vi "Set Backpressure.vi"(6 "Direction":T1, 7 "init":bool, 8 "error in (no error)":errorcluster, 11 "Stand in":refnum<class "Stand.lvclass">) -> (0 "error out":errorcluster, 2 "done":bool, 3 "Stand out":refnum<class "Stand.lvclass">)   [LabVIEW 2019, in "Stand.lvclass"]
uses:
  Stand.lvclass
  D:/GIT H4000/H4000/src/Device_class/Device.lvclass
  TypeDef/Direction.ctl
  TypeDef/SP_TYPE.ctl
  Stand.lvclass/Stand.ctl
  TypeDef/State - BackPressure.ctl
  Valve Mode.ctl
  Device_class/Device.lvclass/Device.ctl
  AI_class/AI.lvclass/AI.ctl
  AnalogComparator_class/AnalogComparator.lvclass/AnalogComparator.ctl
  FPGA/TypeDef/DO index.ctl
  628d624b-520a-41e0-a7db-5fb9c9a9f1d4.vi
  Valve State Mode.vi
  AnalogComparator_class/GetStatus.vi
  Valve State Mode.vi/810e184e-eeb6-4027-a8ae-1422f3ce3d45.vi
  Valve State Mode.vi/57bd4a65-f3dc-44f5-8d68-677c2a197570.vi
  Valve State Mode.vi/03b2f9e4-fceb-4725-9b90-3fd10082a088.vi
  Valve State Mode.vi/3d0d09bd-48e8-482f-b1e2-a36b2bb65234.vi
  Valve State Mode.vi/33d3f26a-dc4a-4f56-bf0a-61d04c5d7434.vi
  Valve State Mode.vi/52af9d47-24d1-4057-80bf-8d93bfb3d17d.vi
  Valve State Mode.vi/094228cb-a119-423c-9af8-5a16f059a318.vi
  Valve State Mode.vi/bf5ad1e6-a0ae-4579-ad74-ca8f304cb7cf.vi
  Valve State Mode.vi/eb4d2b76-f0f0-4e1d-bda0-609c5f37b4e7.vi
  Const All Valve.vi
  Global/Global Constant.vi
  FPGA_API_class/FPGA API.lvclass
  Device_class/Device.lvclass
  AI_class/AI.lvclass
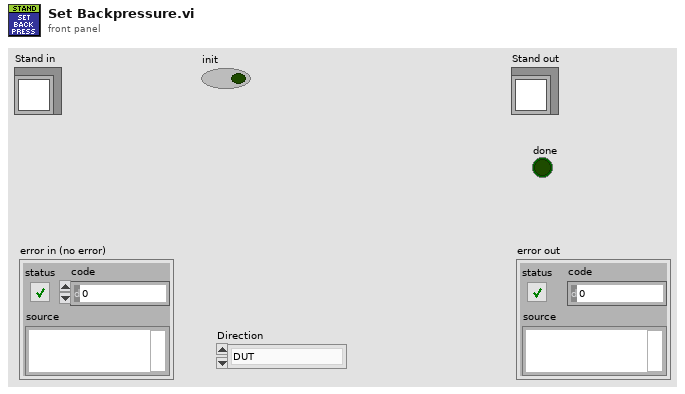
[diagram p1: front panel]
types:
  T1 = typedef "Direction.ctl" = enum8{"DUT", "Chamber"}
  T2 = typedef "SP_TYPE.ctl" = enum16{"ERROR", "ZIRO", "BASE", "SP"}
  T3 = typedef "State - BackPressure.ctl" = enum16{"Check", "Close Inlet", "Open 33_7", "Open Inlet", "Wait", "Close Inlet 2"}
  T4 = typedef "Valve Mode.ctl" = enum16{"Filling DUT", "Filling Chamber", "Pump Pressure DUT", "Pump Pressure Chamber", "Haskel Pressure DUT", "Haskel Pressure Chamber", "Slow Release DUT", "Slow Release Chamber", "Fast Release DUT", "Fast Release Chamber", "Fast Release DUT and Chamber", "Leak Pressure DUT", "Leak Pressure Chamber", "Back Pressure DUT", "Back Pressure Chamber", "Fully Closed", "Drain", "Block DUT", "Block Chamber"}
  T5 = typedef "DO index.ctl" = u8
  T6 = typedef "AI_Data.ctl" = cluster{"Stat Data":T7, "OutOfRangeMax":bool, "OutOfRangeMin":bool, "HIHI":bool, "HI":bool, "LO":bool, "LOLO":bool}
  T7 = typedef "AI Statistics Data.ctl" = cluster{"raw mean":dbl, "scl mean":dbl, "raw mean 1Hz":dbl, "scl mean 1Hz":dbl}
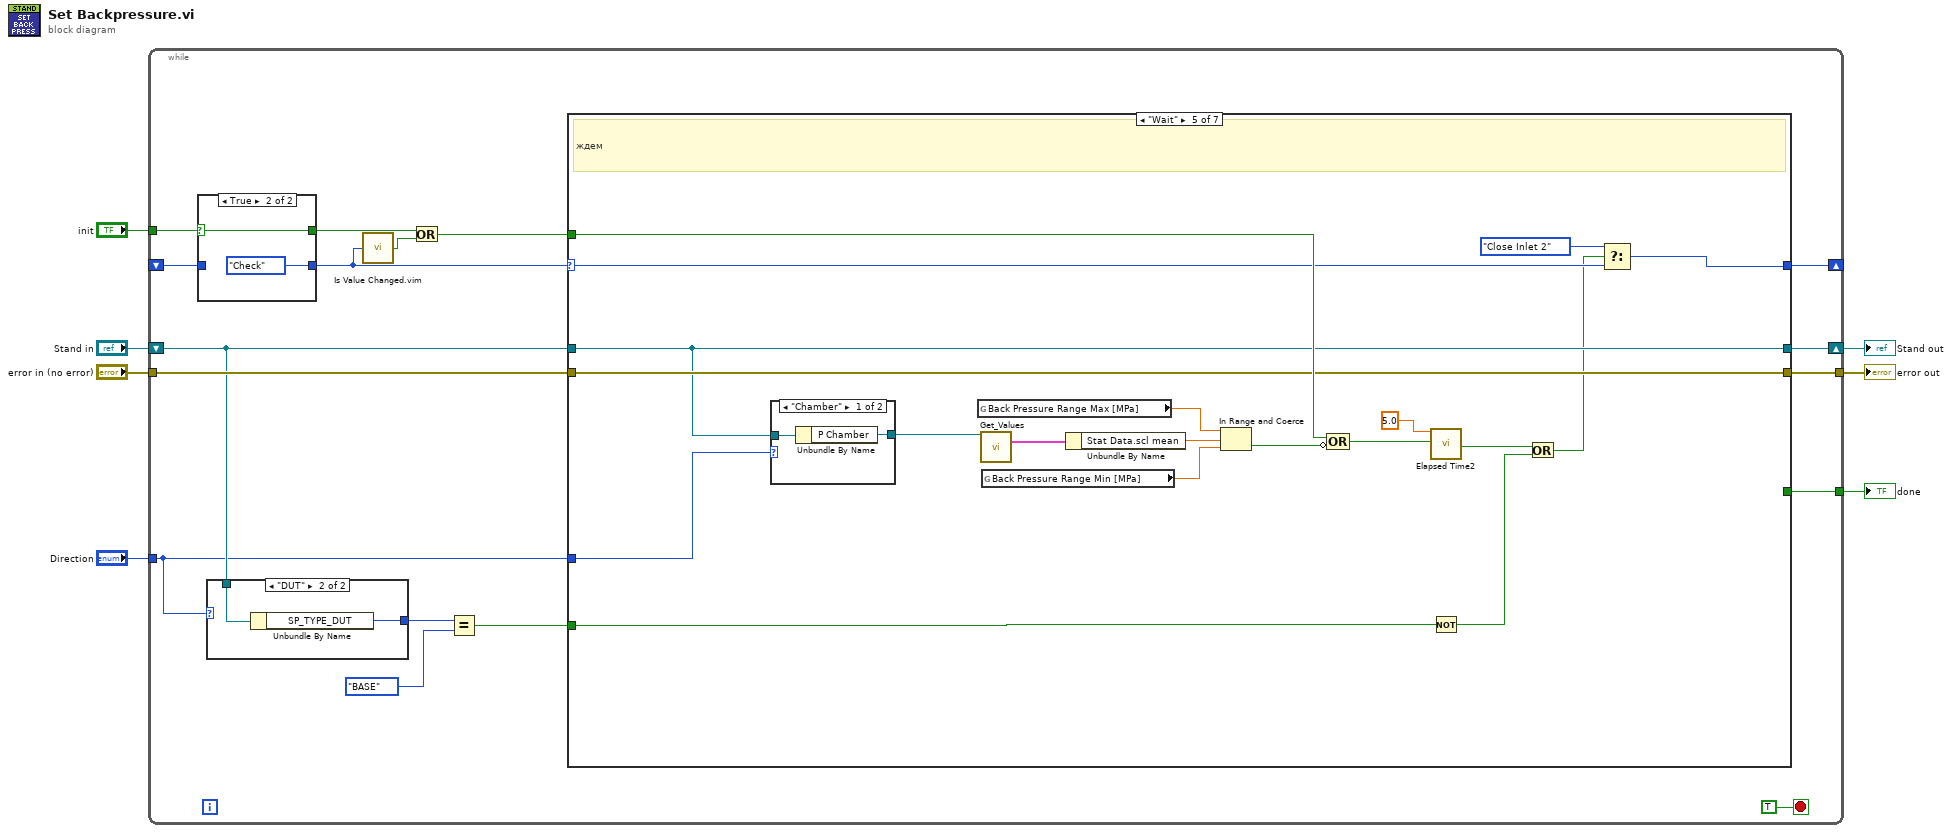
[diagram p0: block diagram]
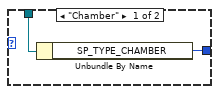
[diagram p2: hidden frame]
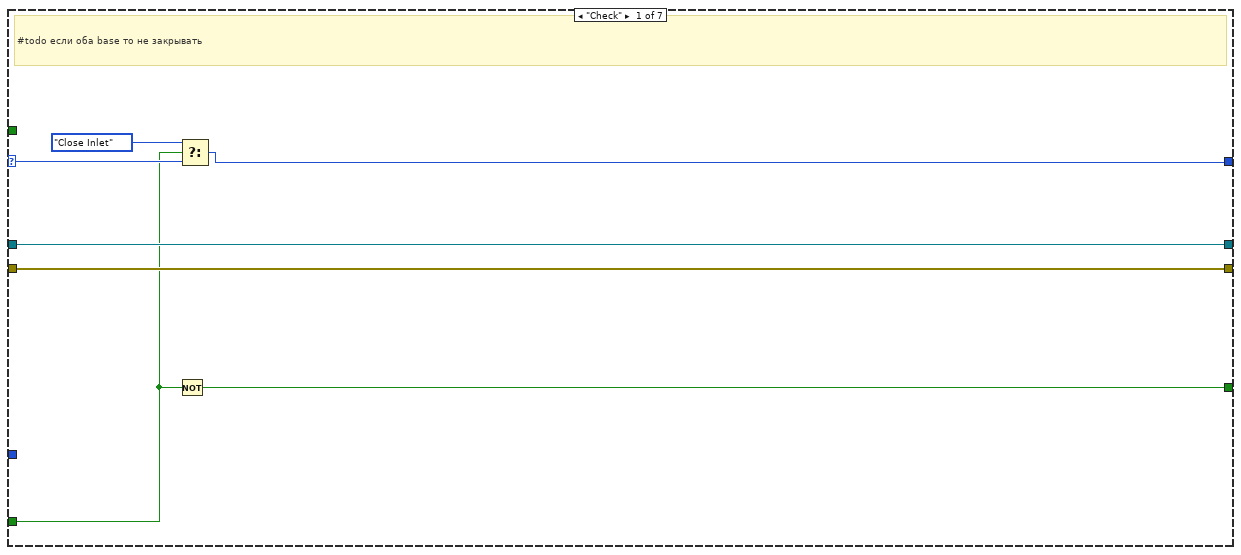
[diagram p4: hidden frame]
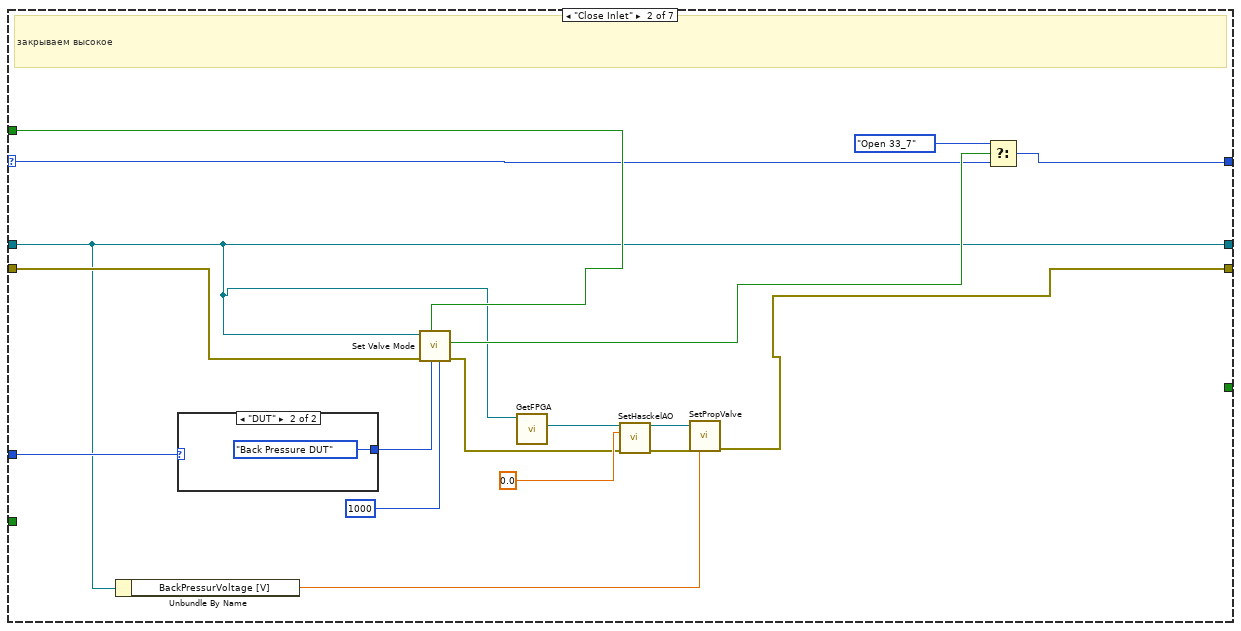
[diagram p5: hidden frame]
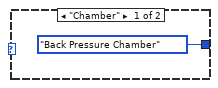
[diagram p6: hidden frame]
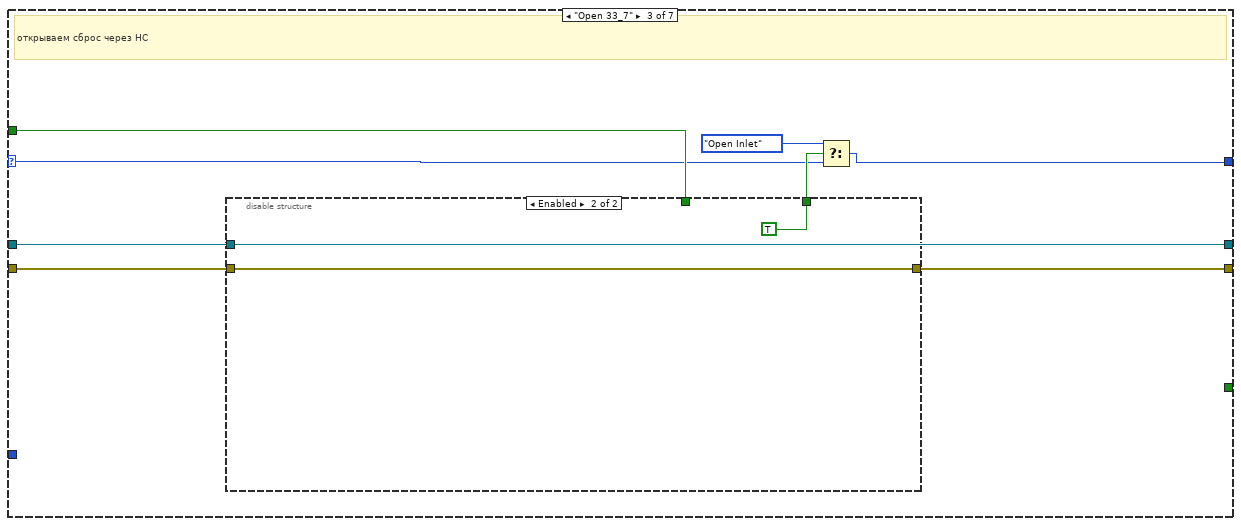
[diagram p7: hidden frame]
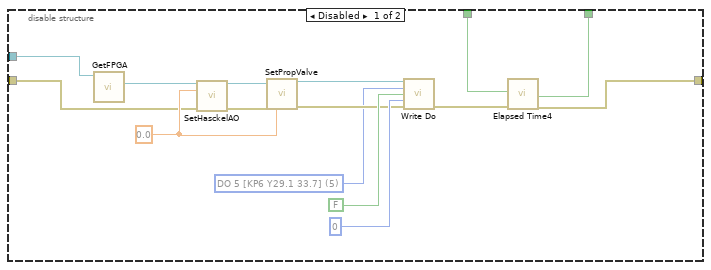
[diagram p8: hidden frame]
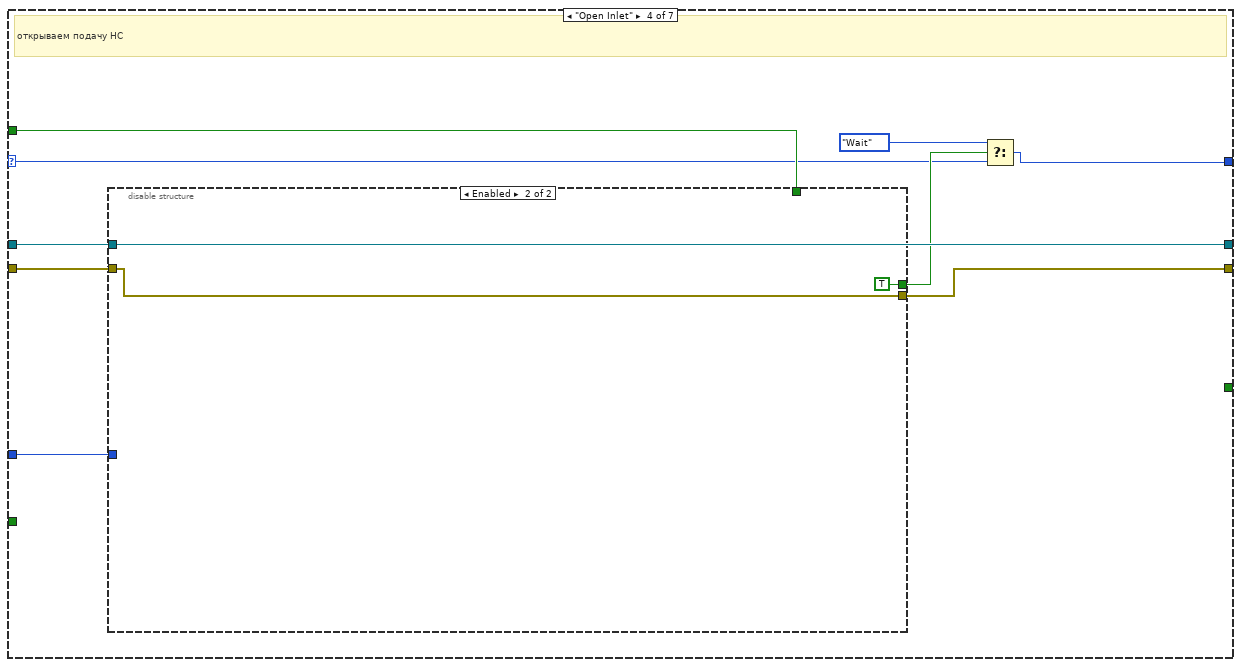
[diagram p9: hidden frame]
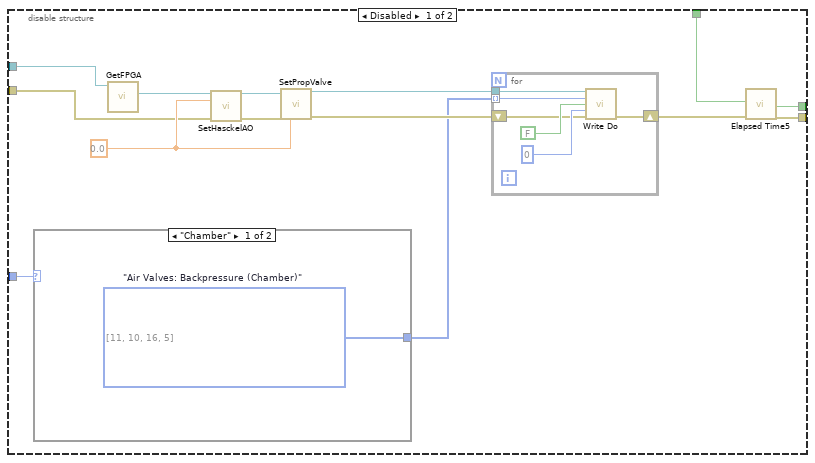
[diagram p10: hidden frame]
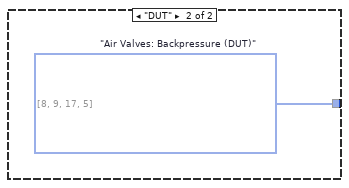
[diagram p11: hidden frame]
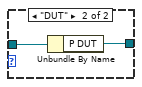
[diagram p12: hidden frame]
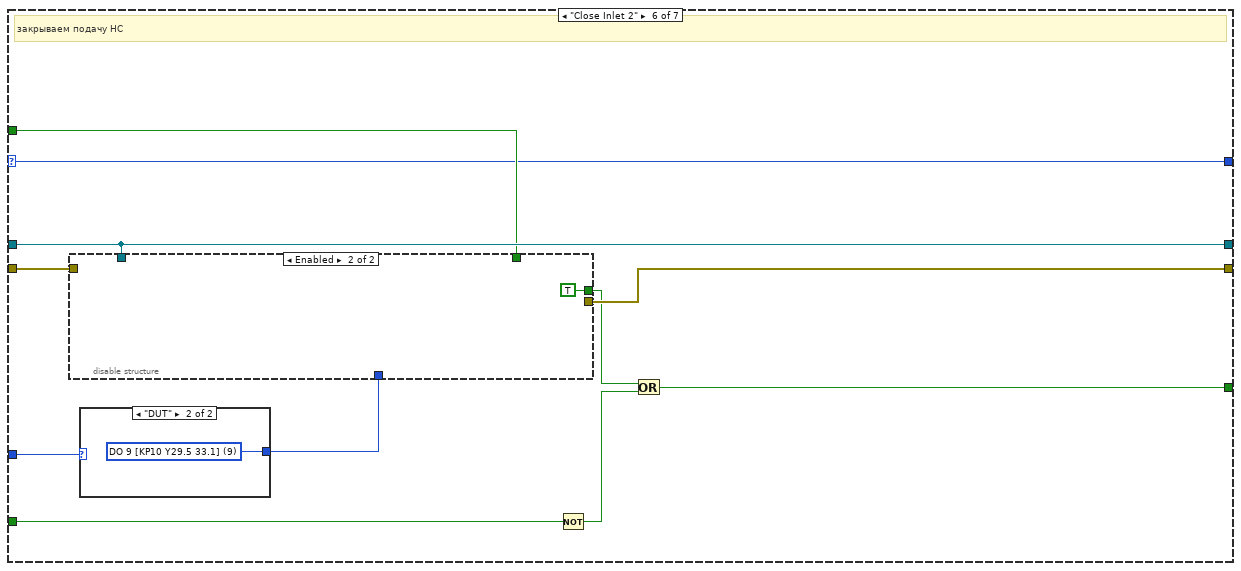
[diagram p13: hidden frame]
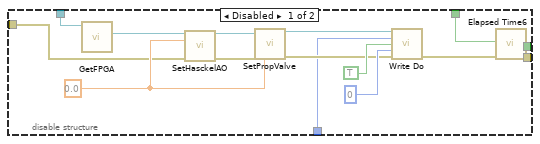
[diagram p14: hidden frame]
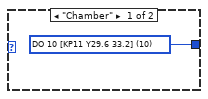
[diagram p15: hidden frame]
diagram:
  n1 = while {
    tunnel: [w24] -> w6
    tunnel: [w23] -> w5
    tunnel: "Direction" -> [w9]
    shift-right: [w13] -> w7
    shift-left: "Stand in" -> [w10]
    tunnel: "init" -> [w18]
    shift-right: [w21] -> _
    shift-left: _ -> [w19]
    tunnel: "error in (no error)" -> [w20]
    stop <- TRUE stop-if-true
    n2 = case shown="True" w18 {
      selector: w18 -> [w29 w32]
      tunnel: [w30 State_-_BackPressure."Check"] -> w16
      tunnel: w19 -> [w30 _]
      tunnel: [w29 w32] -> w17
      frame False {
      }
      frame True {
      }
    }
    n3 = case shown="\"DUT\"" w9 {
      tunnel: w10 -> [w26 w28]
      tunnel: [w25 w27] -> w12
      frame "Chamber" {
        n4 = Unbundle By Name(w26) -> ("SP_TYPE_CHAMBER"=w25:T2)
      }
      frame "DUT" {
        n5 = Unbundle By Name(w28) -> ("SP_TYPE_DUT"=w27:T2)
      }
    }
    n6 = call "Is Value Changed.vim"("value"=w16) -> ("changed or first call?"=w15:bool)
    n7 = Or(x=w17, y=w15) -> (x .or. y?=w14:bool)
    n8 = Equal?(x=w12, y=SP_TYPE."BASE") -> (x = y?=w8:bool)
    n9 = case shown="\"Wait\"" w16 {
      selector: w16 -> [w37 w50 w60 w85 w129 w144 w170]
      tunnel: [w39 w41 w64 w90 w122 w149 w171] -> w13
      tunnel: [w38 w53 w63 w88 w132 w146 w169] -> w24
      tunnel: [w33 _ _ _ _ w142 _] -> w23
      tunnel: w9 -> [_ w54 _ w89 w121 w147 _]
      tunnel: w10 -> [w39 w41 w64 w90 w122 w149 w171]
      tunnel: w20 -> [w38 w56 w66 w92 w132 w150 w169]
      tunnel: w14 -> [_ w52 w62 w87 w135 w145 _]
      tunnel: [w35 w55 w65 w91 w130 w144 w170] -> w21
      tunnel: w8 -> [w34 _ _ _ w118 w141 _]
      frame "Check" {
        # "#todo если оба base то не закрывать"
        n10 = Not(x=w34) -> (.not. x?=w33:bool)
        n11 = Select(t=State_-_BackPressure."Close Inlet", s=w34, f=w37) -> (s? t:f=w35:T3)
      }
      frame "Close Inlet" {
        # "закрываем высокое"
        n12 = Unbundle By Name(w41) -> ("BackPressurVoltage [V]"=w40:dbl)
        n13 = case shown="\"DUT\"" w54 {
          tunnel: [Valve_Mode."Back Pressure Chamber" ("Valve DIR") Valve_Mode."Back Pressure DUT" ("Valve DIR")] -> w48
          frame "Chamber" {
          }
          frame "DUT" {
          }
        }
        n14 = call "Set Valve Mode.vi"("time after close"=u32 1000, "Valve DIR"=w48, "init"=w52, "error in (no error)"=w56, "Stand in"=w41) -> ("error out"=w42:errorcluster, "Done"=w51:bool)  [unwired: 5 in]
        n15 = call "GetFPGA.vi"("Device in"=w41) -> ("FPGA API.lvclass"=w44:refnum<class "FPGA API.lvclass">)  [unwired: 10 in]
        n16 = call-dynamic "SetHasckelAO.vi"("FPGA API in"=w44, "Haskel in"=0.0, "error in (no error)"=w42) -> ("FPGA API out"=w46:refnum<class "FPGA API.lvclass">, "error out"=w45:errorcluster)  [unwired: 11 in]
        n17 = call-dynamic "SetPropValve.vi"("FPGA API in"=w46, "error in (no error)"=w45, "AO 1"=w40) -> ("error out"=w53:errorcluster)  [unwired: 11 in, 1 out]
        n18 = Select(t=State_-_BackPressure."Open 33_7", s=w51, f=w50) -> (s? t:f=w55:T3)
      }
      frame "Open 33_7" {
        # "открываем сброс через НС"
        n19 = disable-structure shown="Enabled" {
          disable-tunnel: w66 -> [w77 w82]
          disable-tunnel: w64 -> [w72 _]
          disable-tunnel: [w69 w82] -> w63
          disable-tunnel: w62 -> [w68 _]
          disable-tunnel: [w67 TRUE ("Time has Elapsed")] -> w61
          frame Disabled {
            w71 = T5 5 items=["DO 0 [KP1] [M12]", "DO 1 [ON KP2] [M21]", "DO 2 [ON KP3] [M24]", "DO 3 [WATER Y18.1 [DO3]]", "DO 4 [WATER Y18.2 [DO4]]", "DO 5 [KP6 Y29.1 33.7]", "DO 6 [KP7 Y29.2 33.8]", "DO 7 [KP8 Y29.3 33.9]", "DO 8 [KP9 Y29.4  33.12]", "DO 9 [KP10 Y29.5 33.1]", "DO 10 [KP11 Y29.6 33.2]", "DO 11 [KP12 Y29.7  33.13]", "DO 12 [KP13 Y29.8  33.11]", "DO 13 [KP14 Y29.9 33.10]", "DO 14 [KP15 Y29.10  33.6]", "DO 15 [KP16 Y29.11  33.5]", "DO 16 [KP17 Y29.12  33.4]", "DO 17 [KP18 Y29.13 33.3]", "DO 18 [AIR KP19]", "DO 19 [STEP DRIVE EN KP20]", "DO 20 [KP21 Y44.1 OPEN]", "DO 21 [ KP22 Y44.1 CLOSE]", "DO 22 [ KP23 Y44.2 OPEN]", "DO 23", "DO 24 [STEP DRIVE 1]", "DO 25 [STEP DRIVE 2]"] ("#DO")
            w78 = 0.0 ("Haskel in")
            n20 = call "GetFPGA.vi"("Device in"=w72) -> ("FPGA API.lvclass"=w81:refnum<class "FPGA API.lvclass">)  [unwired: 10 in]
            n21 = call-dynamic "SetHasckelAO.vi"("FPGA API in"=w81, "Haskel in"=w78, "error in (no error)"=w77) -> ("FPGA API out"=w79:refnum<class "FPGA API.lvclass">, "error out"=w80:errorcluster)  [unwired: 11 in]
            n22 = call-dynamic "SetPropValve.vi"("FPGA API in"=w79, "error in (no error)"=w80, "AO 1"=w78) -> ("FPGA API out"=w74:refnum<class "FPGA API.lvclass">, "error out"=w73:errorcluster)  [unwired: 11 in]
            n23 = call-dynamic "Write Do.vi"("FPGA API in"=w74, "#DO"=w71, "value"=FALSE, "Time uSec"=u32 0, "error in (no error)"=w73) -> ("error out"=w70:errorcluster)  [unwired: 9 in, 1 out]
            n24 = call "Elapsed Time4"("Reset"=w68, "error in (no error)"=w70) -> ("Time has Elapsed"=w67:bool, "error out"=w69:errorcluster)  [unwired: 10 in, 6 out]
          }
          frame Enabled {
          }
        }
        n25 = Select(t=State_-_BackPressure."Open Inlet", s=w61, f=w60) -> (s? t:f=w65:T3)
      }
      frame "Open Inlet" {
        # "открываем подачу НС"
        n26 = disable-structure shown="Enabled" {
          disable-tunnel: w92 -> [w102 w116]
          disable-tunnel: w90 -> [w99 _]
          disable-tunnel: w89 -> [w97 _]
          disable-tunnel: [w95 w116] -> w88
          disable-tunnel: w87 -> [w94 _]
          disable-tunnel: [w93 TRUE ("Time has Elapsed")] -> w86
          frame Disabled {
            w103 = 0.0 ("Haskel in")
            n27 = case shown="\"Chamber\"" w97 {
              tunnel: [w113 w114] -> w98
              frame "Chamber" {
                w113 = T5[] [11, 10, 16, 5] items=["DO 0 [KP1] [M12]", "DO 1 [ON KP2] [M21]", "DO 2 [ON KP3] [M24]", "DO 3 [WATER Y18.1 [DO3]]", "DO 4 [WATER Y18.2 [DO4]]", "DO 5 [KP6 Y29.1 33.7]", "DO 6 [KP7 Y29.2 33.8]", "DO 7 [KP8 Y29.3 33.9]", "DO 8 [KP9 Y29.4  33.12]", "DO 9 [KP10 Y29.5 33.1]", "DO 10 [KP11 Y29.6 33.2]", "DO 11 [KP12 Y29.7  33.13]", "DO 12 [KP13 Y29.8  33.11]", "DO 13 [KP14 Y29.9 33.10]", "DO 14 [KP15 Y29.10  33.6]", "DO 15 [KP16 Y29.11  33.5]", "DO 16 [KP17 Y29.12  33.4]", "DO 17 [KP18 Y29.13 33.3]", "DO 18 [AIR KP19]", "DO 19 [STEP DRIVE EN KP20]", "DO 20 [KP21 Y44.1 OPEN]", "DO 21 [ KP22 Y44.1 CLOSE]", "DO 22 [ KP23 Y44.2 OPEN]", "DO 23", "DO 24 [STEP DRIVE 1]", "DO 25 [STEP DRIVE 2]"]  # "Air Valves: Backpressure (Chamber)"
              }
              frame "DUT" {
                w114 = T5[] [8, 9, 17, 5] items=["DO 0 [KP1] [M12]", "DO 1 [ON KP2] [M21]", "DO 2 [ON KP3] [M24]", "DO 3 [WATER Y18.1 [DO3]]", "DO 4 [WATER Y18.2 [DO4]]", "DO 5 [KP6 Y29.1 33.7]", "DO 6 [KP7 Y29.2 33.8]", "DO 7 [KP8 Y29.3 33.9]", "DO 8 [KP9 Y29.4  33.12]", "DO 9 [KP10 Y29.5 33.1]", "DO 10 [KP11 Y29.6 33.2]", "DO 11 [KP12 Y29.7  33.13]", "DO 12 [KP13 Y29.8  33.11]", "DO 13 [KP14 Y29.9 33.10]", "DO 14 [KP15 Y29.10  33.6]", "DO 15 [KP16 Y29.11  33.5]", "DO 16 [KP17 Y29.12  33.4]", "DO 17 [KP18 Y29.13 33.3]", "DO 18 [AIR KP19]", "DO 19 [STEP DRIVE EN KP20]", "DO 20 [KP21 Y44.1 OPEN]", "DO 21 [ KP22 Y44.1 CLOSE]", "DO 22 [ KP23 Y44.2 OPEN]", "DO 23", "DO 24 [STEP DRIVE 1]", "DO 25 [STEP DRIVE 2]"]  # "Air Valves: Backpressure (DUT)"
              }
            }
            n28 = call "GetFPGA.vi"("Device in"=w99) -> ("FPGA API.lvclass"=w106:refnum<class "FPGA API.lvclass">)  [unwired: 10 in]
            n29 = call-dynamic "SetHasckelAO.vi"("FPGA API in"=w106, "Haskel in"=w103, "error in (no error)"=w102) -> ("FPGA API out"=w104:refnum<class "FPGA API.lvclass">, "error out"=w105:errorcluster)  [unwired: 11 in]
            n30 = call-dynamic "SetPropValve.vi"("FPGA API in"=w104, "error in (no error)"=w105, "AO 1"=w103) -> ("FPGA API out"=w101:refnum<class "FPGA API.lvclass">, "error out"=w100:errorcluster)  [unwired: 11 in]
            n31 = for {
              tunnel: w101 -> [w110]
              tunnel: w98 -> [w108] mode=indexing
              shift-right: [w107] -> w96
              shift-left: w100 -> [w109]
              n32 = call-dynamic "Write Do.vi"("FPGA API in"=w110, "#DO"=w108, "value"=FALSE, "Time uSec"=u32 0, "error in (no error)"=w109) -> ("error out"=w107:errorcluster)  [unwired: 9 in, 1 out]
            }
            n33 = call "Elapsed Time5"("Reset"=w94, "error in (no error)"=w96) -> ("Time has Elapsed"=w93:bool, "error out"=w95:errorcluster)  [unwired: 10 in, 6 out]
          }
          frame Enabled {
          }
        }
        n34 = Select(t=State_-_BackPressure."Wait", s=w86, f=w85) -> (s? t:f=w91:T3)
      }
      frame "Wait" {
        # "ждем"
        n35 = case shown="\"Chamber\"" w121 {
          tunnel: [w137 w139] -> w126
          tunnel: w122 -> [w136 w138]
          frame "Chamber" {
            n36 = Unbundle By Name(w136) -> ("P Chamber"=w137:refnum<class "AI.lvclass">)
          }
          frame "DUT" {
            n37 = Unbundle By Name(w138) -> ("P DUT"=w139:refnum<class "AI.lvclass">)
          }
        }
        n38 = global read "Global Constant.vi" "Back Pressure Range Max [MPa]"() -> (w125:dbl)
        n39 = call "Get_Values.vi"("reference in"=w126) -> ("Data"=w128:T6)  [unwired: 14 in]
        n40 = global read "Global Constant.vi" "Back Pressure Range Min [MPa]"() -> (w124:dbl)
        n41 = Unbundle By Name(w128) -> ("Stat Data.scl mean"=w127:dbl)
        n42 = In Range and Coerce(upper limit=w125, x=w127, lower limit=w124) -> (In Range?=w123:bool)  [unwired: 1 out]
        n43 = Compound Arithmetic op=OR(w135, invert w123) -> (w134:bool)
        n44 = call "Elapsed Time2"("Time Target (s)"=5.0, "Reset"=w134) -> ("Time has Elapsed"=w131:bool)  [unwired: 10 in, 7 out]
        n45 = Not(x=w118) -> (.not. x?=w117:bool)
        n46 = Or(x=w131, y=w117) -> (x .or. y?=w119:bool)
        n47 = Select(t=State_-_BackPressure."Close Inlet 2", s=w119, f=w129) -> (s? t:f=w130:T3)
      }
      frame "Close Inlet 2" {
        # "закрываем подачу НС"
        n48 = case shown="\"DUT\"" w147 {
          tunnel: [w167 w168] -> w148
          frame "Chamber" {
            w167 = T5 10 items=["DO 0 [KP1] [M12]", "DO 1 [ON KP2] [M21]", "DO 2 [ON KP3] [M24]", "DO 3 [WATER Y18.1 [DO3]]", "DO 4 [WATER Y18.2 [DO4]]", "DO 5 [KP6 Y29.1 33.7]", "DO 6 [KP7 Y29.2 33.8]", "DO 7 [KP8 Y29.3 33.9]", "DO 8 [KP9 Y29.4  33.12]", "DO 9 [KP10 Y29.5 33.1]", "DO 10 [KP11 Y29.6 33.2]", "DO 11 [KP12 Y29.7  33.13]", "DO 12 [KP13 Y29.8  33.11]", "DO 13 [KP14 Y29.9 33.10]", "DO 14 [KP15 Y29.10  33.6]", "DO 15 [KP16 Y29.11  33.5]", "DO 16 [KP17 Y29.12  33.4]", "DO 17 [KP18 Y29.13 33.3]", "DO 18 [AIR KP19]", "DO 19 [STEP DRIVE EN KP20]", "DO 20 [KP21 Y44.1 OPEN]", "DO 21 [ KP22 Y44.1 CLOSE]", "DO 22 [ KP23 Y44.2 OPEN]", "DO 23", "DO 24 [STEP DRIVE 1]", "DO 25 [STEP DRIVE 2]"] ("#DO")
          }
          frame "DUT" {
            w168 = T5 9 items=["DO 0 [KP1] [M12]", "DO 1 [ON KP2] [M21]", "DO 2 [ON KP3] [M24]", "DO 3 [WATER Y18.1 [DO3]]", "DO 4 [WATER Y18.2 [DO4]]", "DO 5 [KP6 Y29.1 33.7]", "DO 6 [KP7 Y29.2 33.8]", "DO 7 [KP8 Y29.3 33.9]", "DO 8 [KP9 Y29.4  33.12]", "DO 9 [KP10 Y29.5 33.1]", "DO 10 [KP11 Y29.6 33.2]", "DO 11 [KP12 Y29.7  33.13]", "DO 12 [KP13 Y29.8  33.11]", "DO 13 [KP14 Y29.9 33.10]", "DO 14 [KP15 Y29.10  33.6]", "DO 15 [KP16 Y29.11  33.5]", "DO 16 [KP17 Y29.12  33.4]", "DO 17 [KP18 Y29.13 33.3]", "DO 18 [AIR KP19]", "DO 19 [STEP DRIVE EN KP20]", "DO 20 [KP21 Y44.1 OPEN]", "DO 21 [ KP22 Y44.1 CLOSE]", "DO 22 [ KP23 Y44.2 OPEN]", "DO 23", "DO 24 [STEP DRIVE 1]", "DO 25 [STEP DRIVE 2]"] ("#DO")
          }
        }
        n49 = disable-structure shown="Enabled" {
          disable-tunnel: w150 -> [w161 _]
          disable-tunnel: w149 -> [w156 _]
          disable-tunnel: w148 -> [w155 _]
          disable-tunnel: [w153 _] -> w146
          disable-tunnel: w145 -> [w152 _]
          disable-tunnel: [w151 TRUE ("Time has Elapsed")] -> w143
          frame Disabled {
            w162 = 0.0 ("Haskel in")
            n50 = call "GetFPGA.vi"("Device in"=w156) -> ("FPGA API.lvclass"=w165:refnum<class "FPGA API.lvclass">)  [unwired: 10 in]
            n51 = call-dynamic "SetHasckelAO.vi"("FPGA API in"=w165, "Haskel in"=w162, "error in (no error)"=w161) -> ("FPGA API out"=w163:refnum<class "FPGA API.lvclass">, "error out"=w164:errorcluster)  [unwired: 11 in]
            n52 = call-dynamic "SetPropValve.vi"("FPGA API in"=w163, "error in (no error)"=w164, "AO 1"=w162) -> ("FPGA API out"=w158:refnum<class "FPGA API.lvclass">, "error out"=w157:errorcluster)  [unwired: 11 in]
            n53 = call-dynamic "Write Do.vi"("FPGA API in"=w158, "#DO"=w155, "value"=TRUE, "Time uSec"=u32 0, "error in (no error)"=w157) -> ("error out"=w154:errorcluster)  [unwired: 9 in, 1 out]
            n54 = call "Elapsed Time6"("Reset"=w152, "error in (no error)"=w154) -> ("Time has Elapsed"=w151:bool, "error out"=w153:errorcluster)  [unwired: 10 in, 6 out]
          }
          frame Enabled {
          }
        }
        n55 = Not(x=w141) -> (.not. x?=w140:bool)
        n56 = Or(x=w143, y=w140) -> (x .or. y?=w142:bool)
      }
      frame Default {
      }
    }
  }
  "Stand out" <- w7
  "error out" <- w6
  "done" <- w5
